vi "CtrlRemoveHandler.vi"(0 "Type":T1=enum."Value Change", 1 "Ctrl":refnum<vi>, 2 "Structure":refnum<vi>) -> ()   [LabVIEW 2014]
uses:
  <vilib>/event_ctls.llb/lveventtype.ctl
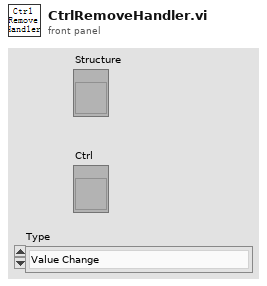
[diagram p1: front panel]
types:
  T1 = typedef "lveventtype.ctl" = enum32{"Null", "Timeout", "Annotation Menu Selection", "Annotation Menu Selection?", "App Instance Close", "App Instance Close?", "Autoscale Range Change", "Bookmark Info Change", "Cell Edit", "Cell Edit?", "Cursor Grab", "Cursor Grab?", "Cursor Menu Selection", "Cursor Menu Selection?", "Cursor Move", "Cursor Release", "Data Change", "Direction Change", "Display State Change", "Drag Ended", "Drag Enter", "Drag Leave", "Drag Over", "Drag Source Update", "Drag Starting", "Drag Starting?", "Drop", "Exec State Change", "Key Down", "Key Down?", "Key Repeat", "Key Repeat?", "Key Up", "Listbox Double Click", "Menu Activation?", "Menu Selection (App)", "Menu Selection? (App)", "Menu Selection (User)", "Mouse Down", "Mouse Down?", "Mouse Enter", "Mouse Leave", "Mouse Move", "Mouse Up", "Mouse Wheel", "NI Security User Change (App)", "Pane Size", "Panel Close", "Panel Close?", "Panel Resize", "Plot Attribute Change", "Scale Range Change", "Shortcut Menu Activation?", "Shortcut Menu Selection (App)", "Shortcut Menu Selection? (App)", "Shortcut Menu Selection (User)", "Tree Double Click", "Tree Drag", "Tree Drag?", "Tree Drop", "Tree Drop?", "Tree Item Close", "Tree Item Close?", "Tree Item Open", "Tree Item Open?", "User Event", "Value Change"}
  T2 = cluster{"Event Type":T1, "Reference":refnum<vi>, "Limit (-1=none)":i32, "Lock Panel?":bool}[]
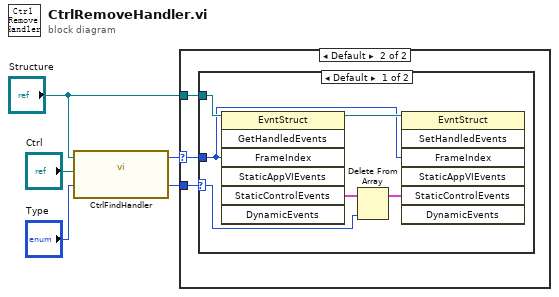
[diagram p0: block diagram]
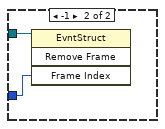
[diagram p3: hidden frame]
diagram:
  n1 = call "CtrlFindHandler.vi"("Type"="Type", "Ctrl"="Ctrl", "Structure"="Structure") -> ("Index"=w1:i32, "Frame"=w3:i32)  [unwired: 1 out]
  n2 = case shown="Default" w3 {
    selector: w3 -> [_ w6]
    tunnel: "Structure" -> [_ w7]
    tunnel: w1 -> [_ w8]
    frame -1 {
    }
    frame Default {
      n3 = case shown="Default" w8 {
        selector: w8 -> [w12 _]
        tunnel: w6 -> [w9 w16]
        tunnel: w7 -> [w14 w15]
        frame Default {
          n4 = invoke class="EvntStruct" method="GetHandledEvents"(reference=w14, "FrameIndex"=w9) -> (reference out=w10:refnum<vi>, "StaticControlEvents"=w13:T2)  [unwired: 5 in, 5 out]
          n5 = Delete From Array(array=w13, index=w12) -> (array with subset deleted=w11:T2)  [unwired: 1 in, 1 out]
          n6 = invoke class="EvntStruct" method="SetHandledEvents"(reference=w10, "FrameIndex"=w9, "StaticControlEvents"=w11) -> ()  [unwired: 4 in, 7 out]
        }
        frame -1 {
          n7 = invoke class="EvntStruct" method="Remove Frame"(reference=w15, "Frame Index"=w16) -> ()  [unwired: 2 in, 4 out]
        }
      }
    }
  }
